vi "test_Add Waveform Output Channels.vi"(8 "error in (no error)":errorcluster, 11 "TestCase in":refnum<class "FPGA Addon Adding Channel Items Unit Tests.lvclass">) -> (0 "error out":errorcluster, 3 "TestCase out":refnum<class "FPGA Addon Adding Channel Items Unit Tests.lvclass">)   [LabVIEW 2020, in "FPGA Addon Adding Channel Items Unit Tests.lvclass"]
uses:
  FPGA Addon Adding Channel Items Unit Tests.lvclass
  <vilib>/NI VeriStand/Custom Device API/Custom Device Channel.ctl
  <vilib>/NI VeriStand/Custom Device API/Custom Device Channel Type.ctl
  Addon/Addon System Explorer/Types/Channel Type.ctl
  Addon/Addon System Explorer/Types/SE UI Cluster.ctl
  <vilib>/NI VeriStand/Custom Device API/Custom Device Item Ref.ctl
  FPGA Addon Adding Channel Items Unit Tests.lvclass/FPGA Addon Adding Channel Items Unit Tests.ctl
  Addon/Addon Shared/SubVIs/Constants.vi
  <vilib>/NI VeriStand/Custom Device Tools/Custom Device Utility Library/NI VeriStand - Search for Item by GUID.vi
  <vilib>/NI/NI VeriStand Advanced SysDef API/_SubVIs/SysDef.Search.GUIDs.vi
  <vilib>/addons/_JKI Toolkits/VI Tester/TestCase.llb/TestCase.lvclass
  Addon/Addon System Explorer/FPGA Addon System Explorer.lvlib
  <vilib>/NI VeriStand/Custom Device Tools/Custom Device Utility Library/Custom Device Utility Library.lvlib
  Addon/Addon Shared/FPGA Addon Shared.lvlib
  <vilib>/NI/NI VeriStand Advanced SysDef API/SysDef API/Advanced System Definition.lvlib
  <vilib>/NI VeriStand/Custom Device API/Custom Device API.lvlib
  C:/Program Files (x86)/National Instruments/LabVIEW 2020/vi.lib/addons/_JKI Toolkits/VI Tester/TestCase.llb/TestCase.lvclass
panel:
  out "GUIDs":string[](array[string])
  out "Channels":T1[](array[typedef])
  in  "remove":bool
  in  "add":bool
  out "Names":string[](array[string])
  in  "Available Registers":i32[](listbox)
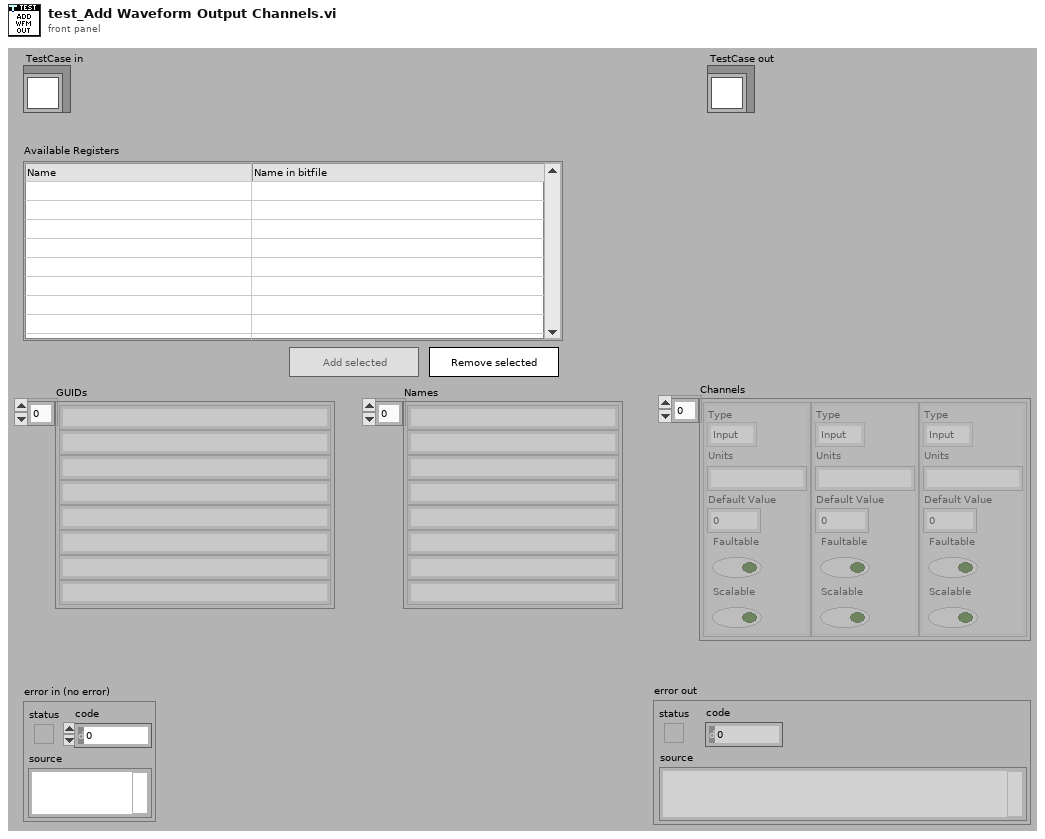
[diagram p1: front panel]
types:
  T1 = typedef "Custom Device API.lvlib/Custom Device Channel.ctl" = cluster{"Type":T2, "Units":string, "Default Value":dbl, "Faultable":bool, "Scalable":bool}
  T2 = typedef "Custom Device API.lvlib/Custom Device Channel Type.ctl" = enum16{"Input", "Output"}
  T3 = typedef "FPGA Addon System Explorer.lvlib/SE UI Cluster.ctl" = cluster{"Node Ptr":T4, "Add":refnum<vi>, "Remove":refnum<vi>, "Registers ListBox":refnum<vi>}
  T4 = typedef "Custom Device API.lvlib/Custom Device Item Ref.ctl" = u64
  T5 = typedef "FPGA Addon System Explorer.lvlib/Channel Type.ctl" = enum16{"Write Channel", "Read Channel", "Write Waveform", "Read Waveform"}
  T6 = typedef "Advanced System Definition.lvlib/TreeItem.Info.ctl" = cluster{"Name":string, "Description":string, "GUID":string, "Is Channel":bool, "Channel":T1, "Is Waveform":bool, "Waveform":T7}
  T7 = typedef "Custom Device API.lvlib/Custom Device Waveform.ctl" = cluster{"Data Type":T8, "Units":string}
  T8 = typedef "Custom Device API.lvlib/Custom Device Waveform DataType.ctl" = enum16{"Double", "Complex Double"}
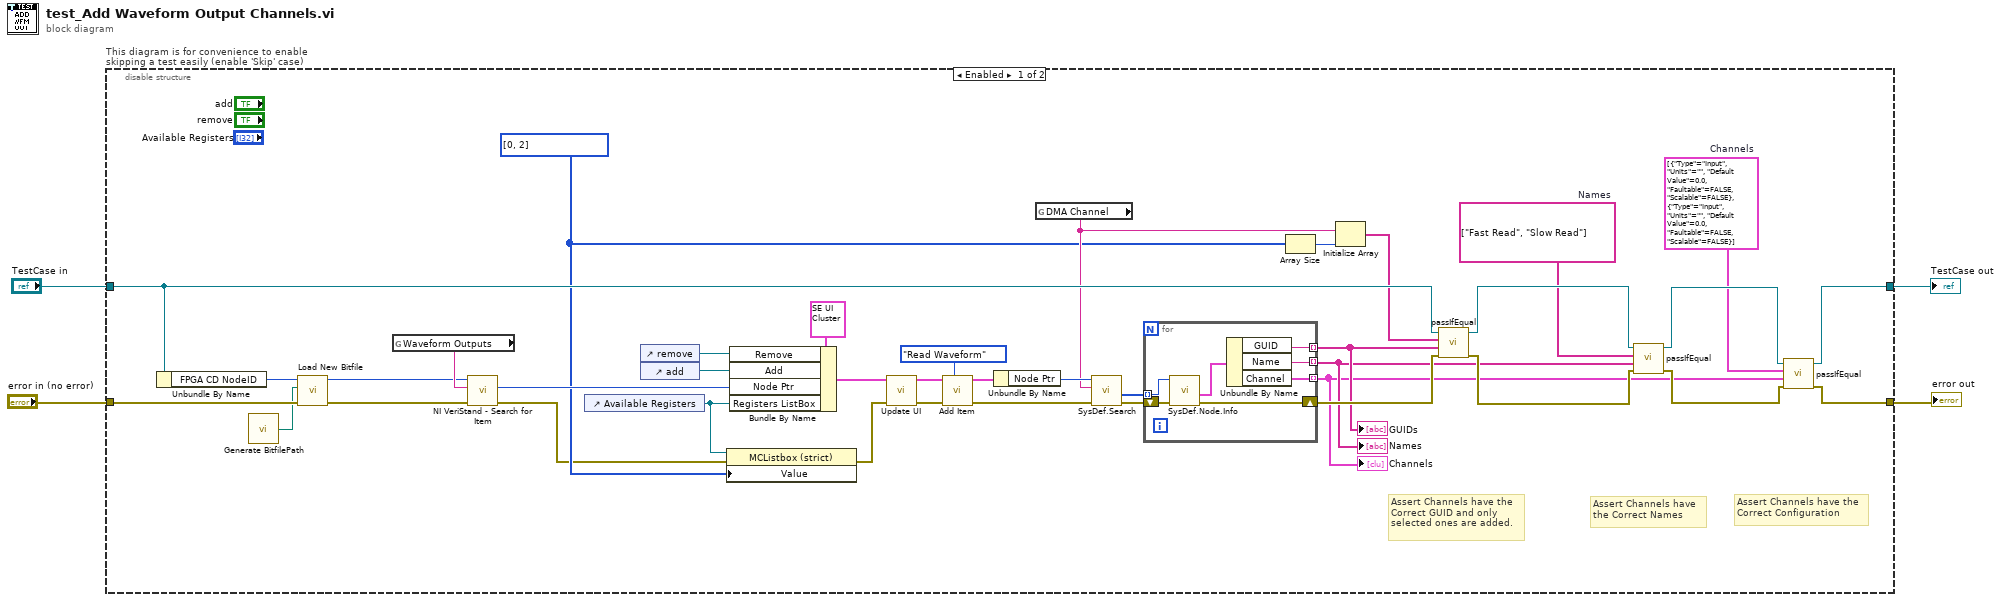
[diagram p0: block diagram]
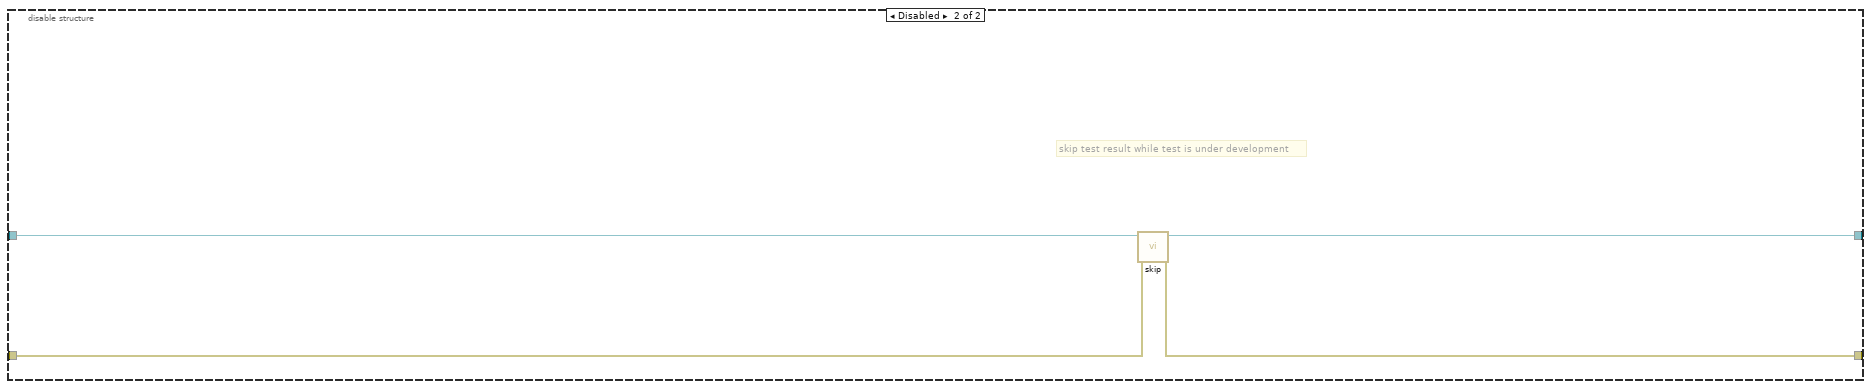
[diagram p2: hidden frame]
diagram:
  n1 = disable-structure "This diagram is for convenience to enable skipping a test easily (enable 'Skip' case)" shown="Enabled" {
    disable-tunnel: "TestCase in" -> [w35 w54]
    disable-tunnel: [w31 w52] -> w1
    disable-tunnel: [w28 w53] -> w3
    disable-tunnel: "error in (no error)" -> [w25 w51]
    frame Enabled {
      w27 = T1[] [{"Type"=enum."Input", "Units"="", "Default Value"=0.0, "Faultable"=FALSE, "Scalable"=FALSE}, {"Type"=enum."Input", "Units"="", "Default Value"=0.0, "Faultable"=FALSE, "Scalable"=FALSE}]  # Channels
      w32 = string[] ["Fast Read", "Slow Read"]  # Names
      w7 = i32[] [0, 2] ("selected")
      # "Assert Channels have the Correct Configuration"
      # "Assert Channels have the Correct Names"
      # "Assert Channels have the Correct GUID and only selected ones are added."
      n2 = Unbundle By Name(w35) -> ("FPGA CD NodeID"=w24:u64)
      n3 = call "Generate BitfilePath.vi"() -> ("Bitfile path"=w23:path)
      n4 = call "Load New Bitfile.vi"("error in (no error)"=w25, "NewVal"=w23, "Item Ref in"=w24) -> ("error out"=w26:errorcluster, "Section Ref out"=w18:T4)  [unwired: 7 in]
      n5 = global read "Constants.vi" "Waveform Outputs"() -> (w42:string)
      n6 = call-poly <vilib>:"NI VeriStand - Search for Item.vi"("error in"=w26, "Item GUID"=w42, "Section Ref in"=w18) -> ("error out"=w6:errorcluster, "Item Ref"=w12:T4)  [unwired: 5 in, 2 out]
      n7 = control-ref of="Available Registers"() -> (w8:refnum<vi>)
      n8 = control-ref of="remove"() -> (w11:refnum<vi>)
      n9 = control-ref of="add"() -> (w10:refnum<vi>)
      n10 = property class="MCListbox (strict)"(reference=w8, error in=w6, "Value"=w7) -> (error out=w5:errorcluster)  [unwired: 1 out]
      n11 = Bundle By Name(cluster=T3 {"Node Ptr"=18446744073709551615, "Add"=refnum, "Remove"=refnum, "Registers ListBox"=refnum} ("SE UI cluster in"), "Remove"=w11, "Add"=w10, "Node Ptr"=w12, "Registers ListBox"=w8) -> (w9:T3)
      n12 = call "Update UI.vi"("error in (no error)"=w5, "SE UI cluster in"=w9) -> ("error out"=w15:errorcluster, "SE UI cluster out"=w14:T3)  [unwired: 8 in]
      n13 = call "Add Item.vi"("Action"=Channel_Type."Read Waveform", "error in (no error)"=w15, "SE UI cluster in"=w14) -> ("error out"=w17:errorcluster, "SE UI cluster out"=w22:T3)  [unwired: 7 in]
      n14 = Unbundle By Name(w22) -> ("Node Ptr"=w40:T4)
      n15 = global read "Constants.vi" "DMA Channel"() -> (w20:string)
      n16 = call-poly <vilib>:"SysDef.Search.vi"("error in (no error)"=w17, "GUID"=w20, "nodeID"=w40) -> ("error out"=w41:errorcluster, "Values Out"=w39:u64[])  [unwired: 5 in, 2 out]
      n17 = for {
        tunnel: w39 -> [w47] mode=indexing
        tunnel: [w45] -> w33 mode=indexing
        tunnel: [w44] -> w16 mode=indexing
        tunnel: [w46] -> w36 mode=indexing
        shift-right: [w49] -> w37
        shift-left: w41 -> [w50]
        n18 = call <vilib>:"SysDef.Node.Info.vi"("error in (no error)"=w50, "nodeID"=w47) -> ("error out"=w49:errorcluster, "Item Info"=w48:T6)  [unwired: 6 in, 2 out]
        n19 = Unbundle By Name(w48) -> ("GUID"=w46:string, "Name"=w45:string, "Channel"=w44:T1)
      }
      "Names" <- w33
      "Channels" <- w16
      "GUIDs" <- w36
      n20 = Array Size(array=w7) -> (size(s)=w19:i32)
      n21 = Initialize Array(w20, w19) -> (w21:string[])
      n22 = call-dynamic "passIfEqual.vi"("error in (no error)"=w37, "y"=w36, "x"=w21, "TestCase in"=w35) -> ("error out"=w38:errorcluster, "TestCase out"=w34:refnum<class "FPGA Addon Adding Channel Items Unit Tests.lvclass">)  [unwired: 6 in]
      n23 = call-dynamic "passIfEqual.vi"("error in (no error)"=w38, "y"=w33, "x"=w32, "TestCase in"=w34) -> ("error out"=w29:errorcluster, "TestCase out"=w30:refnum<class "FPGA Addon Adding Channel Items Unit Tests.lvclass">)  [unwired: 6 in]
      n24 = call-dynamic "passIfEqual.vi"("error in (no error)"=w29, "y"=w16, "x"=w27, "TestCase in"=w30) -> ("error out"=w28:errorcluster, "TestCase out"=w31:refnum<class "FPGA Addon Adding Channel Items Unit Tests.lvclass">)  [unwired: 6 in]
    }
    frame Disabled {
      # "skip test result while test is under development"
      n25 = call <vilib>:"skip.vi"("error in (no error)"=w51, "TestCase in"=w54) -> ("error out"=w53:errorcluster, "TestCase out"=w52:refnum<class "FPGA Addon Adding Channel Items Unit Tests.lvclass">)  [unwired: 8 in]
    }
  }
  "error out" <- w3
  "TestCase out" <- w1
